vi "MAG INIT.vi"(0 "Queue in":refnum<queue>, 5 "Field Range":T2={"Sweep States"=enum."SET FIELD", "VISA Connection"="COM4", "Fields(T)"=[]}, 7 "SMS VISA resource name IN":refnum<visa-resource-name>, 9 "PSU Status In":T1 {"Trip Current" format="%.3f"; "Trip Field" format="%.4f"; "Voltage" format="%.2f"; "Field Constant" format="%.6f"; "MID Setpoint (T)" format="%.4f"; "MID Setpoint (A)" format="%.3f"; "MAX Setpoint (T)" format="%.4f"; "MAX Setpoint (A)" format="%.3f"; "Heater Voltage" format="%.2f"; "V Limit (V)" format="%.2f"; "Ramp Rate (A/s)" format="%.3f"; "Output (A)" format="%.3f"; "Output (T)" format="%.4f"; "Persistent Current" format="%.3f"; "Persistent Field" format="%.4f"}, 11 "error in (no error)":errorcluster) -> (4 "Queue out":refnum<queue>, 6 "VISA Resource Name Out":refnum<visa-resource-name>, 10 "PSU Status Out":T1 {"Trip Current" format="%.3f"; "Trip Field" format="%.4f"; "Voltage" format="%.2f"; "Field Constant" format="%.6f"; "MID Setpoint (T)" format="%.4f"; "MID Setpoint (A)" format="%.3f"; "MAX Setpoint (T)" format="%.4f"; "MAX Setpoint (A)" format="%.3f"; "Heater Voltage" format="%.2f"; "V Limit (V)" format="%.2f"; "Ramp Rate (A/s)" format="%.3f"; "Output (A)" format="%.3f"; "Output (T)" format="%.4f"; "Persistent Current" format="%.3f"; "Persistent Field" format="%.4f"}, 15 "error out":errorcluster)   [LabVIEW 2025]
uses:
  <instrlib>/SMS LabVIEW Drivers/Source Code/Public/PSU Status.ctl
  <instrlib>/SMS LabVIEW Drivers/Source Code/Cryogenic Ltd SMSXXX.lvlib
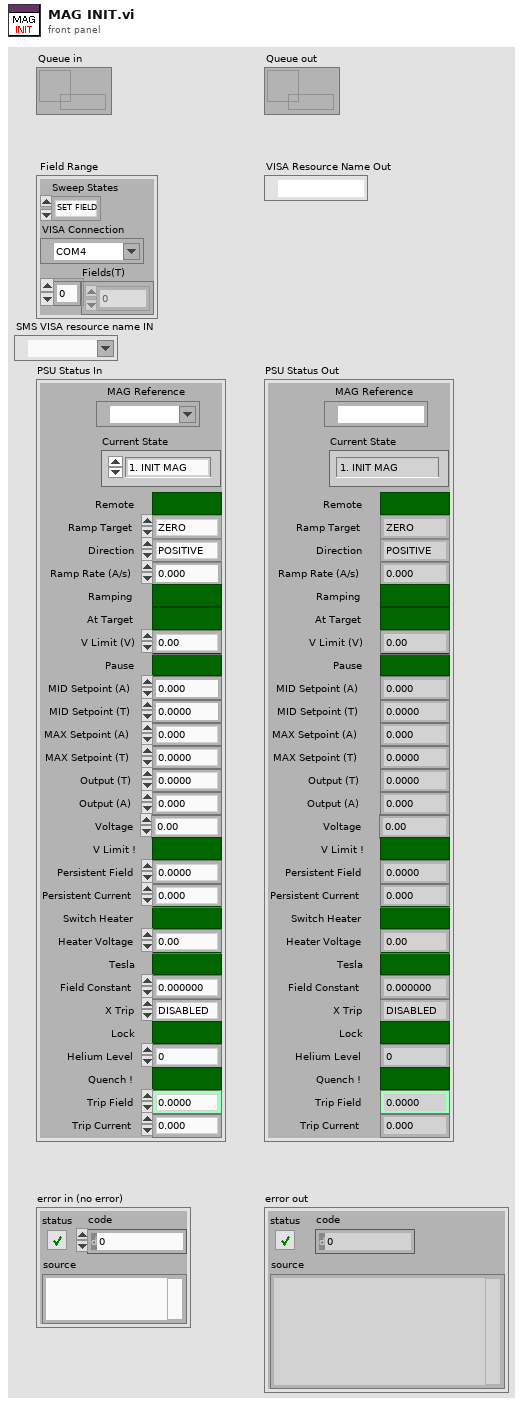
[diagram p1: front panel]
types:
  T1 = typedef "PSU Status.ctl" = cluster{"Ramp Target":enum16{"ZERO", "MID", "MAX"}, "Pause":bool, "Switch Heater":bool, "Persistent Field":dbl, "Persistent Current":dbl, "Tesla":bool, "Output (T)":dbl, "Output (A)":dbl, "X Trip":enum16{"DISABLED", "ENABLED", "ACTIVE"}, "Ramp Rate (A/s)":dbl, "V Limit (V)":dbl, "Heater Voltage":dbl, "MAX Setpoint (A)":dbl, "MAX Setpoint (T)":dbl, "MID Setpoint (A)":dbl, "MID Setpoint (T)":dbl, "Lock":bool, "Field Constant":dbl, "Remote":bool, "Direction":enum16{"POSITIVE", "NEGATIVE", "OPEN", "UNIPOLAR"}, "Helium Level":u16, "Quench !":bool, "Voltage":dbl, "V Limit !":bool, "Ramping":bool, "At Target":bool, "Trip Field":dbl, "Trip Current":dbl, "Current State":enum16{"1. INIT MAG", "2. MAG ON", "3. MAG_STAB", "4. MAG IDLE", "5. PREP NEXT FIELD", "6. APPLY NEXT FIELD", "7. PREP OFF", "8. MAG OFF (Reset)"}, "MAG Reference":refnum<visa-resource-name>}
  T2 = cluster{"Sweep States":enum16{"SET FIELD", "SWEEP IDLE", "NEXT FIELD", "SWEEP DONE"}, "VISA Connection":refnum<visa-resource-name>, "Fields(T)":dbl[]}
  T3 = enum16{"1. INIT MAG", "2. MAG ON", "3. MAG_STAB", "4. MAG IDLE", "5. PREP NEXT FIELD", "6. APPLY NEXT FIELD", "7. PREP OFF", "8. MAG OFF (Reset)"}
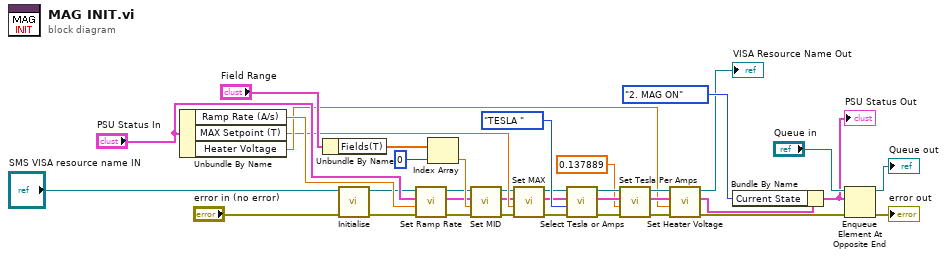
[diagram p0: block diagram]
diagram:
  n1 = Unbundle By Name("PSU Status In") -> ("Ramp Rate (A/s)"=w36:dbl, "MAX Setpoint (T)"=w8:dbl, "Heater Voltage"=w12:dbl)
  n2 = Unbundle By Name("Field Range") -> ("Fields(T)"=w33:dbl[])
  n3 = call <instrlib>:"Initialise.vi"("error in"="error in (no error)", "SMS VISA resource name IN"="SMS VISA resource name IN") -> ("error out"=w19:errorcluster, "VISA Resource Name Out"=w18:refnum<visa-resource-name>)  [unwired: 8 in]
  n4 = call <instrlib>:"Set Ramp Rate.vi"("Error in (no error)"=w19, "Ramp Rate (A/s)"=w36, "PSU Status In"="PSU Status In", "VISA Resource Name In"=w18) -> ("Error out"=w7:errorcluster, "PSU Status Out"=w6:T1, "VISA Resource Name Out"=w5:refnum<visa-resource-name>)  [unwired: 4 in, 1 out]
  n5 = Index Array(array=w33, index=0) -> (element=w35:dbl)
  n6 = call <instrlib>:"Set MID.vi"("Error in (no error)"=w7, "MID (T or A)"=w35, "PSU Status In"=w6, "VISA Resource Name In"=w5) -> ("Error out"=w2:errorcluster, "PSU Status Out"=w3:T1, "VISA Resource Name Out"=w4:refnum<visa-resource-name>)  [unwired: 4 in, 1 out]
  n7 = call <instrlib>:"Set MAX.vi"("Error in (no error)"=w2, "MAX  (T or A)"=w8, "PSU Status In"=w3, "VISA Resource Name In"=w4) -> ("Error out"=w22:errorcluster, "PSU Status Out"=w21:T1, "VISA Resource Name Out"=w20:refnum<visa-resource-name>)  [unwired: 4 in, 1 out]
  n8 = call <instrlib>:"Select Tesla or Amps.vi"("Error in (no error)"=w22, "Tesla/Amps"=enum16{"AMPS", "TESLA "}."TESLA ", "PSU Status In"=w21, "VISA Resource Name In"=w20) -> ("Error out"=w23:errorcluster, "PSU Status Out"=w25:T1, "VISA Resource Name Out"=w24:refnum<visa-resource-name>)  [unwired: 4 in, 1 out]
  n9 = call <instrlib>:"Set Tesla Per Amps.vi"("Error in (no error)"=w23, "Tesla Per Amp"=0.137889, "PSU Status In"=w25, "VISA Resource Name In"=w24) -> ("Error out"=w10:errorcluster, "PSU Status Out"=w15:T1, "VISA Resource Name Out"=w27:refnum<visa-resource-name>)  [unwired: 4 in, 1 out]
  n10 = call <instrlib>:"Set Heater Voltage.vi"("Error in (no error)"=w10, "Heater Voltage (V)"=w12, "PSU Status In"=w15, "VISA Resource Name In"=w27) -> ("Error out"=w31:errorcluster, "PSU Status Out"=w16:T1, "VISA Resource Name Out"=→"VISA Resource Name Out":refnum<visa-resource-name>)  [unwired: 4 in, 1 out]
  n11 = Bundle By Name(cluster=w16, "Current State"=T3."2. MAG ON") -> (w17:T1)
  "PSU Status Out" <- w17
  n12 = Enqueue Element At Opposite End(queue="Queue in", element=w17, error in (no error)=w31) -> (queue out=→"Queue out":refnum<queue>, error out=→"error out":errorcluster)  [unwired: 1 in, 1 out]
